vi "MarbleDispenserMk4.vi"   [LabVIEW 2016]
uses:
  <vilib>/NXT/Block Support/NXT_InputPort.ctl
  <vilib>/NXT/Block Support/NXT_OutputPort.ctl
  <vilib>/NXT/Dual Mode Library/Sensors/Touch_Released.vi
  <vilib>/NXT/NXTIO Xnodes/NXTIONodeSubVIs/NXTStopMotors.vi
  <vilib>/NXT/NXTIO Xnodes/NXTIONodeSubVIs/NXTMoveMotors.vi
  <vilib>/NXT/NXTIO Xnodes/NXTIONodeSubVIs/NXTMotorRunDistance.vi
  <vilib>/NXT/Dual Mode Library/Waits/Wait_Num.vi
  <vilib>/NXT/Dual Mode Library/Sensors/Touch_Pressed.vi
  <vilib>/NXT/Subs/LVHSConnector.ctl
  <vilib>/NXT/NXTIO Xnodes/AddressXNode/NXTIOAddress.xnode
  <vilib>/NXT/NXTIO Xnodes/NXTIOXNode/NXTIO.xnode
  <vilib>/NXT/Dual Mode Library/Sensors/EV3_Color_Reflect.vi
  <vilib>/NXT/LegoClasses/BrickReference/BrickReference.lvclass
types:
  T1 = typedef "NXT_InputPort.ctl" = u32
  T2 = typedef "NXT_OutputPort.ctl" = u8
  T3 = typedef "LVHSConnector.ctl" = refnum<class "BrickReference.lvclass">
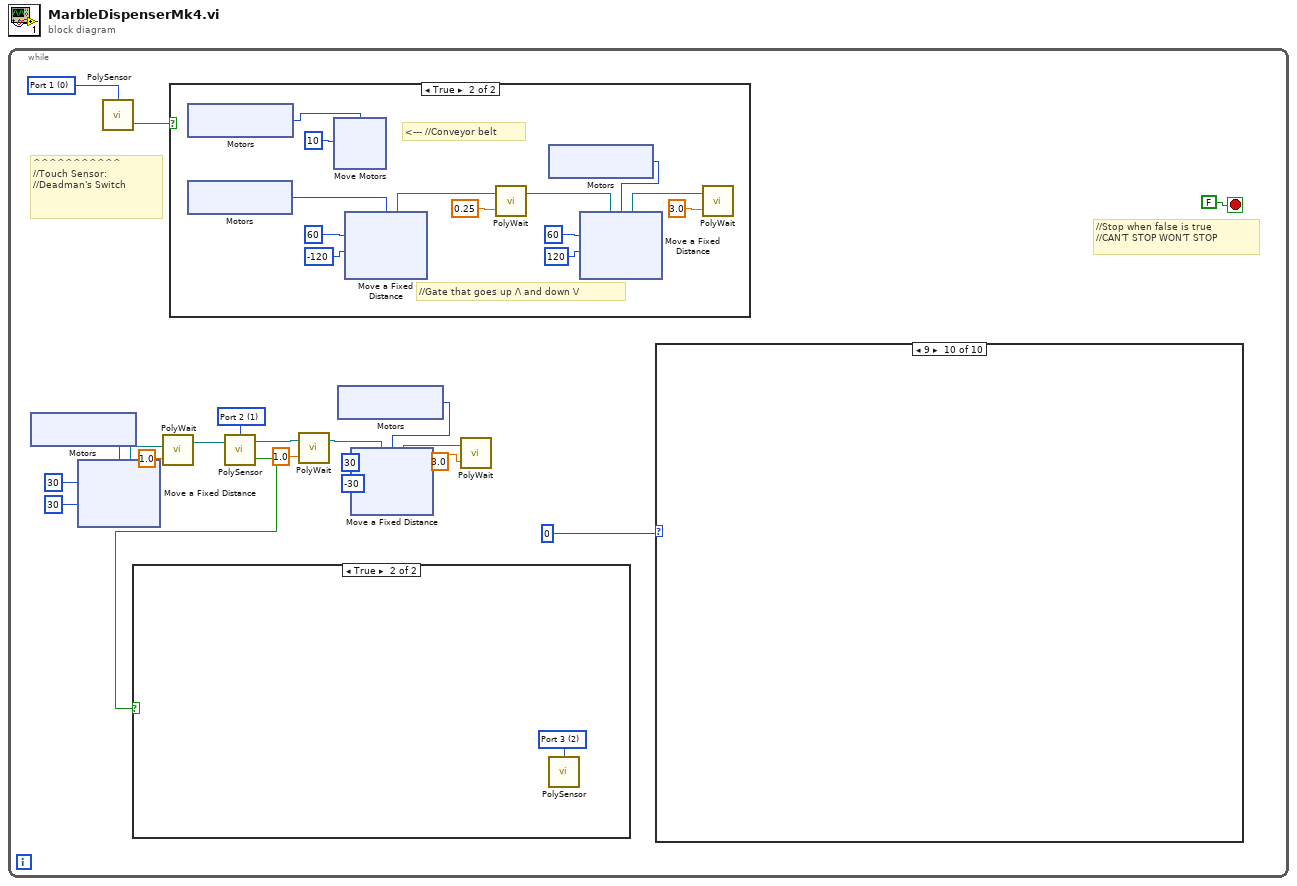
[diagram p0: block diagram]
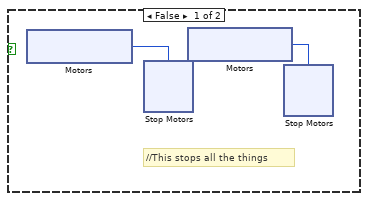
[diagram p12: hidden frame]
diagram:
  n1 = while {
    stop <- FALSE stop-if-true
    w6 = T1 1 items=["Port 1", "Port 2", "Port 3", "Port 4"] ("Port (Port 1)")
    w20 = T1 0 items=["Port 1", "Port 2", "Port 3", "Port 4"] ("Port (Port 1)")
    # "//Stop when false is true\n//CAN'T STOP WON'T STOP"
    # "^^^^^^^^^^^\n//Touch Sensor:\n//Deadman's Switch"
    n2 = xnode "Motors"() -> ("Motor"=w13:T2)
    n3 = xnode "Move a Fixed Distance"("Speed 1"=30, "Distance 1"=30, "Motors"=w13) -> ("NXT/EV3"=w16:T3)  [unwired: 1 in]
    n4 = call-poly <vilib>:"PolySensor.vi"("Port (Port 1)"=w20) -> ("Yes / No"=w18:bool)  [unwired: 2 in, 1 out]
    n5 = call-poly <vilib>:"PolyWait.vi"("Time (1 sec)"=1.0, "NXT/EV3"=w16) -> ("NXT/EV3"=w7:T3)  [unwired: 2 in]
    n6 = case shown="True" w18 {
      frame False {
        # "//This stops all the things"
        n7 = xnode "Motors"() -> ("Motor"=w45:T2)
        n8 = xnode "Stop Motors"("Motors"=w45) -> ()  [unwired: 1 in, 1 out]
        n9 = xnode "Motors"() -> ("Motor"=w44:T2)
        n10 = xnode "Stop Motors"("Motors"=w44) -> ()  [unwired: 1 in, 1 out]
      }
      frame True {
        # "//Gate that goes up /\\ and down \\/"
        # "<--- //Conveyor belt"
        n11 = xnode "Motors"() -> ("Motor"=w70:T2)
        n12 = xnode "Motors"() -> ("Motor"=w64:T2)
        n13 = xnode "Move Motors"("Power/Speed 1"=10, "Motors"=w70) -> ()  [unwired: 1 in, 1 out]
        n14 = xnode "Move a Fixed Distance"("Speed 1"=-120, "Distance 1"=60, "Motors"=w64) -> ("NXT/EV3"=w67:T3)  [unwired: 1 in]
        n15 = call-poly <vilib>:"PolyWait.vi"("Time (1 sec)"=0.25, "NXT/EV3"=w67) -> ("NXT/EV3"=w59:T3)  [unwired: 2 in]
        n16 = xnode "Motors"() -> ("Motor"=w58:T2)
        n17 = xnode "Move a Fixed Distance"("Speed 1"=120, "Distance 1"=60, "Motors"=w58, "NXT/EV3"=w59) -> ("NXT/EV3"=w62:T3)
        n18 = call-poly <vilib>:"PolyWait.vi"("Time (1 sec)"=3.0, "NXT/EV3"=w62) -> ()  [unwired: 2 in, 1 out]
      }
    }
    n19 = call-poly <vilib>:"PolySensor.vi"("NXT/EV3"=w7, "Port (Port 1)"=w6) -> ("Yes / No"=w4:bool, "NXT/EV3"=w3:T3)  [unwired: 1 in]
    n20 = case shown="True" w4 {
      frame False {
      }
      frame True {
        w21 = T1 2 items=["Port 1", "Port 2", "Port 3", "Port 4"] ("Port (Port 1)")
        n21 = call-poly <vilib>:"PolySensor.vi"("Port (Port 1)"=w21) -> ()  [unwired: 2 in, 2 out]
      }
    }
    n22 = call-poly <vilib>:"PolyWait.vi"("Time (1 sec)"=sgl 1.0, "NXT/EV3"=w3) -> ("NXT/EV3"=w2:T3)  [unwired: 2 in]
    n23 = xnode "Motors"() -> ("Motor"=w8:T2)
    n24 = xnode "Move a Fixed Distance"("Speed 1"=-30, "Distance 1"=30, "Motors"=w8, "NXT/EV3"=w2) -> ("NXT/EV3"=w11:T3)
    n25 = call-poly <vilib>:"PolyWait.vi"("Time (1 sec)"=3.0, "NXT/EV3"=w11) -> ()  [unwired: 2 in, 1 out]
    n26 = case shown="9" 0 {
      frame 0, Default {
      }
      frame 1 {
      }
      frame 2 {
      }
      frame 3 {
      }
      frame 4 {
      }
      frame 5 {
      }
      frame 6 {
      }
      frame 7 {
      }
      frame 8 {
      }
      frame 9 {
      }
    }
  }
